vi "Handle Error.vi"(8 "error in (no error)":errorcluster, 11 "CS++BaseActor in":refnum<class "CS++BaseActor.lvclass">) -> (0 "error out":errorcluster, 2 "stop actor?":bool=TRUE, 3 "CS++BaseActor out":refnum<class "CS++BaseActor.lvclass">)   [LabVIEW 2015, in "CS++BaseActor.lvlib" / "CS++BaseActor.lvclass"]
doc: "(<B>Filename</B>: Actor Framework.lvlib:Actor.lvclass:Handle Error.vi)\n\nDefines how the actor handles an error that occurred while processing a message.\n\nBy default, this method does nothing except stop the actor. This method also treats error code 43 (coming from <B>error in</B>) as a sign that the actor shut down normally. In this situation, the Handle Error method does not return the error on <B>error out</B>, meaning the actor's caller will not receive it. All other error codes will be returned on <B>error out</B>.\n\nA descendant class may override this method to change this behavior."
uses:
  CS++BaseActor.lvclass
  CS++BaseActor.lvclass/CS++BaseActor.ctl
  Libraries/Base/Severity.ctl
  <vilib>/Utility/error.llb/DialogType.ctl
  <vilib>/ActorFramework/Actor/Actor.lvclass
  Libraries/Base/CS++Base.lvlib
  Libraries/Utilities/CS++Utilities.lvlib
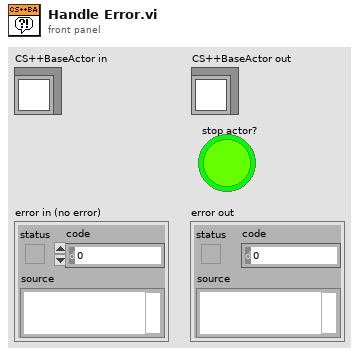
[diagram p1: front panel]
types:
  T1 = typedef "CS++Base.lvlib/Severity.ctl" = enum16{"emergency", "alert", "critical", "error", "warning", "notice", "info", "debug"}
  T2 = typedef "DialogType.ctl" = u16
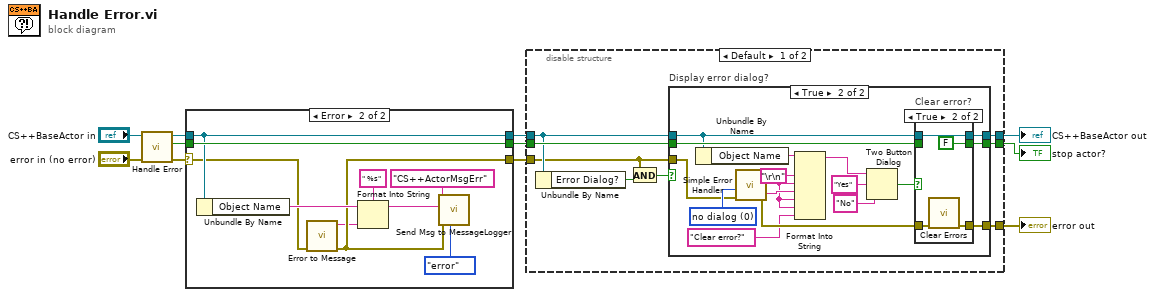
[diagram p0: block diagram]
diagram:
  n1 = call-parent "Handle Error.vi"("error in (no error)"="error in (no error)", "Actor in"="CS++BaseActor in") -> ("error out"=w9:errorcluster, "stop actor?"=w8:bool, "Actor out"=w7:refnum<class "CS++BaseActor.lvclass">)  [unwired: 7 in]
  n2 = case shown="Error" w9 {
    selector: w9 -> [w14 w17]
    tunnel: [w14 w16] -> w1
    tunnel: [w13 w24] -> w4
    tunnel: w8 -> [w13 w24]
    tunnel: [w12 w22] -> w2
    tunnel: w7 -> [w12 w22]
    frame No Error {
    }
    frame Error {
      n3 = Unbundle By Name(w22) -> ("Object Name"=w21:string)
      n4 = call "Error to Message.vi"("Error In"=w17) -> ("Error Out"=w16:errorcluster, "Error Message"=w15:string)  [unwired: 9 in]
      n5 = Format Into String(format string=" %s", initial string=w21, w15) -> (resulting string=w18:string)  [unwired: 1 in, 1 out]
      n6 = call "Send Msg to MessageLogger.vi"("Severity Code (info)"=Severity."error", "Error In"=w16, "Message Content"=w18, "Message Tag"="CS++ActorMsgErr") -> ()  [unwired: 7 in, 1 out]
    }
  }
  n7 = disable-structure shown="Default" {
    disable-tunnel: [w32 w61] -> w6
    disable-tunnel: [w31 w59] -> w5
    disable-tunnel: w4 -> [w30 w60]
    disable-tunnel: [w29 w60] -> w3
    disable-tunnel: w2 -> [w28 w61]
    disable-tunnel: w1 -> [w26 w59]
    frame condition #0 (active) {
      n8 = Unbundle By Name(w28) -> ("Error Dialog?"=w25:bool)
      n9 = And(x=w26, y=w25) -> (x .and. y?=w27:bool)
      n10 = case "Display error dialog?" shown="True" w27 {
        tunnel: w30 -> [w35 w44]
        tunnel: [w33 w49] -> w31
        tunnel: [w35 w43] -> w29
        tunnel: w28 -> [w34 w38]
        tunnel: [w34 w42] -> w32
        tunnel: w26 -> [w33 w37]
        frame False {
        }
        frame True {
          w36 = "\r\n"
          w51 = T2 0 items=["no dialog", "OK message", "continue or stop message", "OK message + warnings", "continue/stop + warnings"] ("type of dialog (OK msg:1)")
          n11 = Unbundle By Name(w38) -> ("Object Name"=w39:string)
          n12 = call <vilib>:"Simple Error Handler.vi"("type of dialog (OK msg:1)"=w51, "error in (no error)"=w37) -> ("error out"=w50:errorcluster, "message"=w41:string)  [unwired: 3 in, 3 out]
          n13 = Format Into String(initial string=w39, w36, w36, w41, w36, w36, "Clear error?" ("input 7")) -> (resulting string=w48:string)  [unwired: 2 in, 1 out]
          n14 = Two Button Dialog(message=w48, 1:"No" ("F button name (\"Cancel\")"), 2:"Yes" ("T button name (\"OK\")")) -> (T button?=w45:bool)
          n15 = case "Clear error?" shown="True" w45 {
            tunnel: w50 -> [w54 w58]
            tunnel: [w54 w57] -> w49
            tunnel: w44 -> [w53 _]
            tunnel: [w53 FALSE ("stop actor?")] -> w43
            tunnel: [w52 w55] -> w42
            tunnel: w38 -> [w52 w55]
            frame False {
            }
            frame True {
              n16 = call <vilib>:"Clear Errors.vi"("error in (no error)"=w58) -> ("error out"=w57:errorcluster)  [unwired: 5 in, 1 out]
            }
          }
        }
      }
    }
    frame condition #1 {
    }
  }
  "CS++BaseActor out" <- w6
  "error out" <- w5
  "stop actor?" <- w3
